vi "state_machine.vi"() -> ()   [LabVIEW 2017, in "DemoSequencer.lvlib"]
uses:
  DemoSequencer.lvlib
  Utilities/WordManipulationLibrary.lvlib
  Utilities/StateMachineStatus.ctl
  Utilities/Bit Manipulation.lvlib
  Utilities/Controlword_Commands.ctl
  Utilities/StateMachine.ctl
panel:
  out "Data Out":u16 format="%08b"
  out "Status":T1
  in  "Device Control Command":T2=enum."Switch On"
  out "Waveform Chart":dbl(graph)
  in  "End Program":bool
  in  "Stop Move":bool
  in  "SLM Velocity":dbl
  in  "SLM Position":dbl
  in  "StraightLineMove":bool
  out "StatusWord":u16
  in  "stop":bool
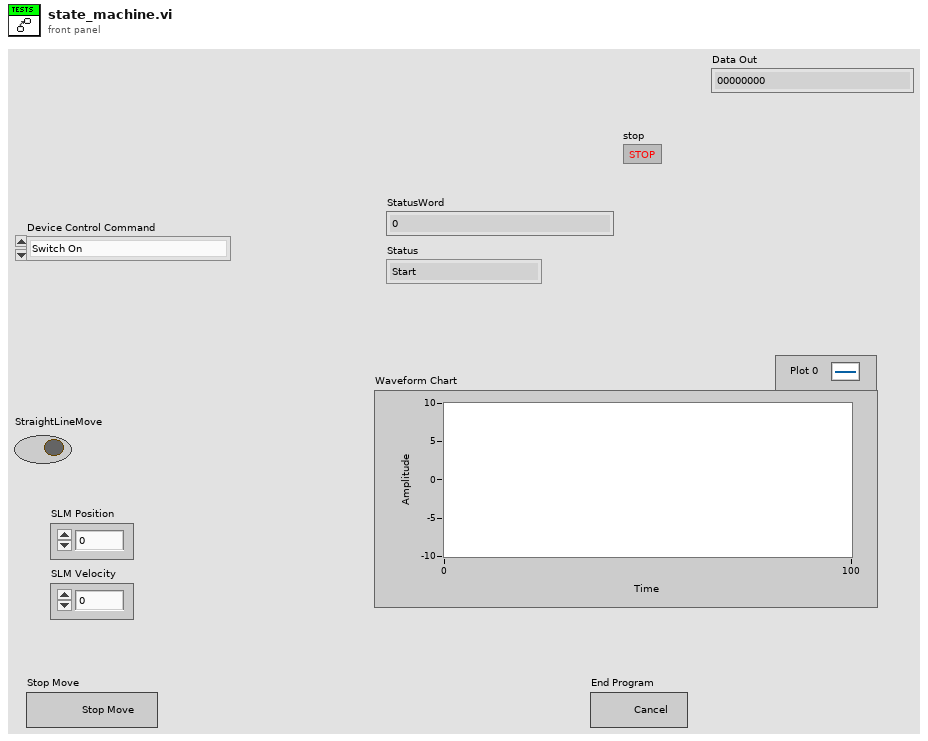
[diagram p1: front panel]
types:
  T1 = typedef "WordManipulationLibrary.lvlib/StateMachine.ctl" = enum16{"Start", "Not Ready to Switch On", "Switch On Disabled", "Ready to Switch On", "Switched On", "Operation enable", "Quick Stop Active", "Fault Reaction Active", "Fault"}
  T2 = typedef "WordManipulationLibrary.lvlib/Controlword_Commands.ctl" = enum16{"Shutdown", "Switch On", "Disable Voltage", "Quick Stop", "Disable Op", "Enable Op", "Fault Reset", "Error"}
  T3 = typedef "StateMachineStatus.ctl" = enum16{"init", "StateMachineManipulation", "waiting", "PreparingMove", "ProcessingMove", "end"}
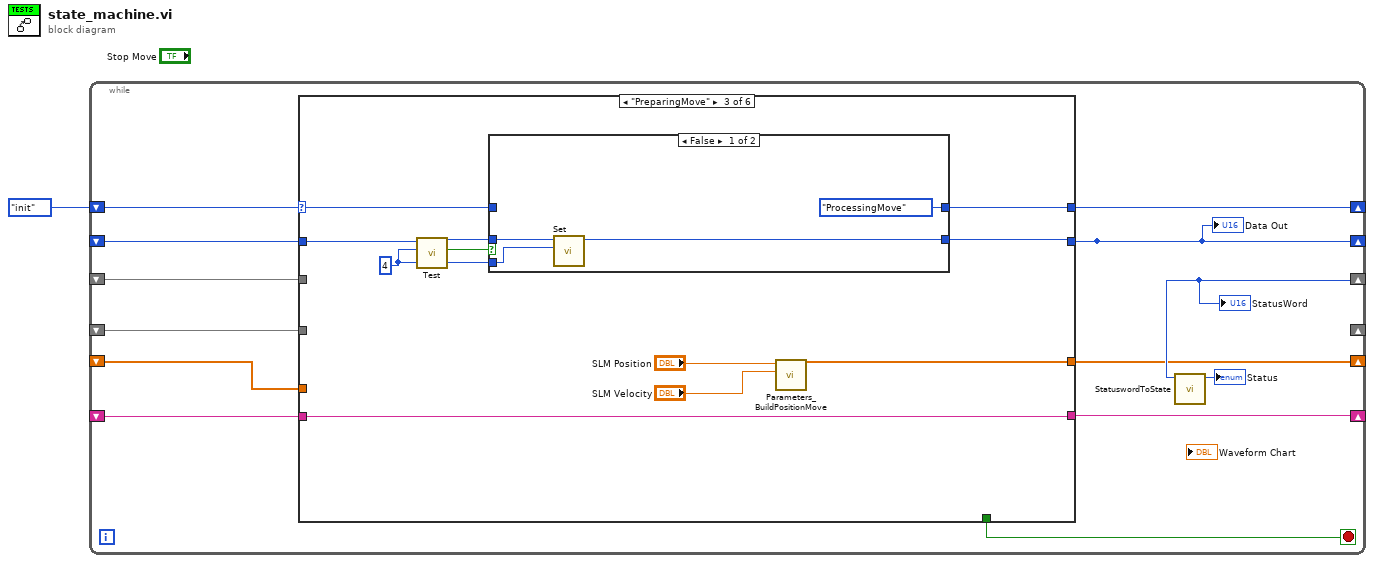
[diagram p0: block diagram]
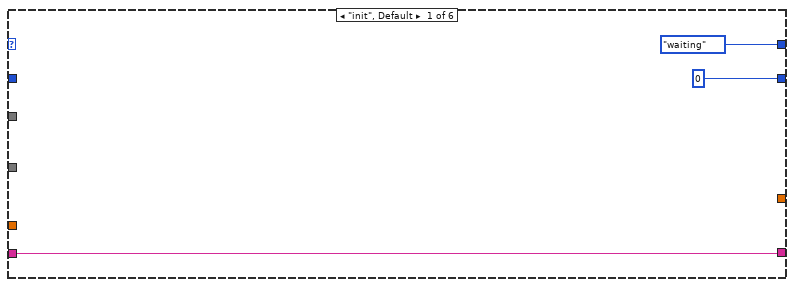
[diagram p2: hidden frame]
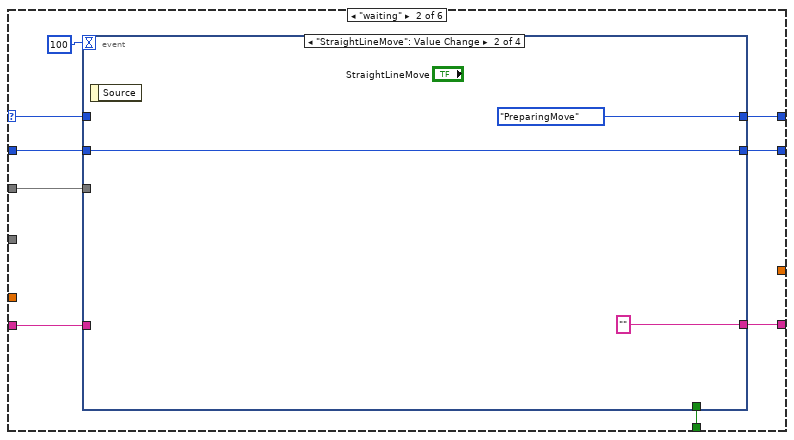
[diagram p3: hidden frame]
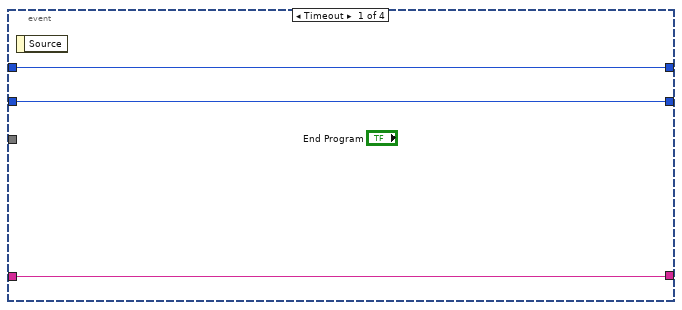
[diagram p4: hidden frame]
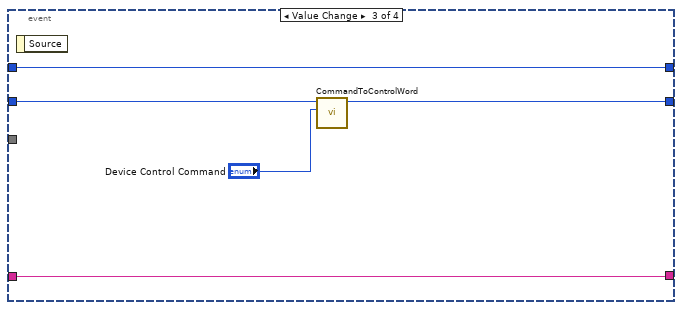
[diagram p5: hidden frame]
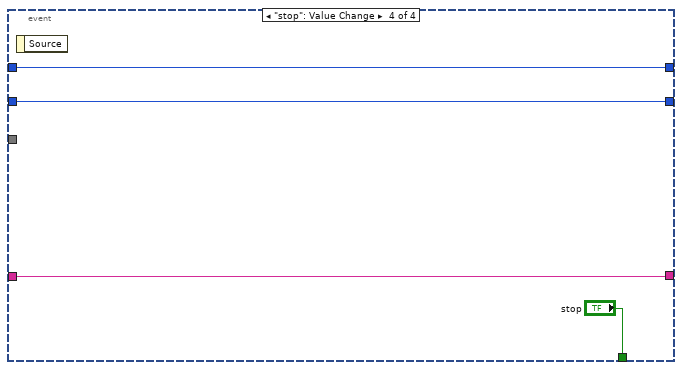
[diagram p6: hidden frame]
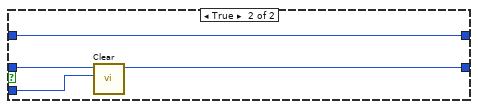
[diagram p7: hidden frame]
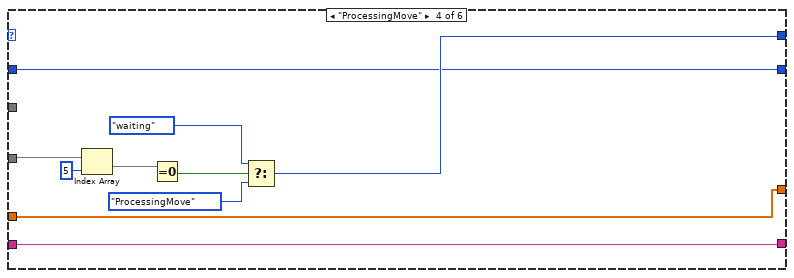
[diagram p8: hidden frame]
diagram:
  n1 = while {
    shift-right: ["StatusWord"] -> _
    shift-left: _ -> [w11]
    shift-right: [w14] -> _
    shift-left: StateMachineStatus."init" -> [w15]
    shift-right: [w13] -> _
    shift-left: _ -> [w12]
    shift-right: [w10] -> _
    shift-left: _ -> [w7]
    shift-right: _ -> [w9]
    shift-left: _ -> [w8]
    shift-right: [w3] -> _
    shift-left: _ -> [w2]
    stop <- w6 stop-if-true
    n2 = case shown="\"PreparingMove\"" w15 {
      selector: w15 -> [_ w23 w47 _ w72 w76]
      tunnel: [u16 0 ("ControlWord") w24 w49 w64 w73 w77] -> w13
      tunnel: [StateMachineStatus."waiting" w22 w48 w65 w72 w76] -> w14
      tunnel: w12 -> [_ w26 w53 w64 w73 w77]
      tunnel: w11 -> [_ w25 _ _ _ _]
      tunnel: [w16 w21 w46 w63 w74 w75] -> w10
      tunnel: [_ _ w43 w62 _ _] -> w3
      tunnel: w8 -> [_ _ _ w71 _ _]
      tunnel: w7 -> [w16 w19 w46 w63 w74 w75]
      tunnel: [_ w20 _ _ _ _] -> w6
      tunnel: w2 -> [_ _ _ w62 _ _]
      frame "init", Default {
      }
      frame "waiting" {
        n3 = event shown="[1] \"StraightLineMove\": Value Change" {
          selector: _ -> [_ _ _ _]
          dyn-events: _ -> [_ _ _ _]
          timeout: 100 -> [_ _ _ _]
          tunnel: w26 -> [w30 w31 w38 w40]
          tunnel: w25 -> [_ _ _ _]
          tunnel: [w30 w31 w36 w40] -> w24
          tunnel: w23 -> [w29 _ w34 w41]
          tunnel: [w29 StateMachineStatus."PreparingMove" w34 w41] -> w22
          tunnel: [w28 "" w35 w39] -> w21
          tunnel: [_ _ _ "stop"] -> w20
          tunnel: w19 -> [w28 _ w35 w39]
          event Timeout {
            n4 = event-data() -> ()  [unwired: 1 in, 1 out]
          }
          event "StraightLineMove": Value Change {
            n5 = event-data() -> ()  [unwired: 1 in, 1 out]
          }
          event Value Change {
            n6 = event-data() -> ()  [unwired: 1 in, 1 out]
            n7 = call "CommandToControlWord.vi"("Device Control Command"="Device Control Command", "ControlWord In"=w38) -> ("ControlWord Out"=w36:u16)  [unwired: 9 in]
          }
          event "stop": Value Change {
            n8 = event-data() -> ()  [unwired: 1 in, 1 out]
          }
        }
      }
      frame "PreparingMove" {
        w50 = u8 4 ("Bit to test")
        n9 = call "Test.vi"("Bit to test"=w50, "Data_In"=w53) -> ("bit value"=w52:bool, "Data_Out"=w51:u16)  [unwired: 8 in]
        n10 = case shown="False" w52 {
          tunnel: w51 -> [w57 w61]
          tunnel: w50 -> [w56 w60]
          tunnel: [w55 w59] -> w49
          tunnel: [StateMachineStatus."ProcessingMove" w58] -> w48
          tunnel: w47 -> [_ w58]
          frame False {
            n11 = call "Set.vi"("Bit to set"=w56, "Data_In"=w57) -> ("Data_Out"=w55:u16)  [unwired: 9 in]
          }
          frame True {
            n12 = call "Clear.vi"("Bit to clear"=w60, "Data_In"=w61) -> ("Data_Out"=w59:u16)  [unwired: 9 in]
          }
        }
        n13 = call "Parameters_BuildPositionMove.vi"("Velocity"="SLM Velocity", "Target Position"="SLM Position") -> ("Parameters"=w43:dbl[])  [unwired: 9 in]
      }
      frame "ProcessingMove" {
        n14 = Index Array(array=w71, index=5) -> (element=w69)
        n15 = Equal To 0?(x=w69) -> (x = 0?=w68:bool)
        n16 = Select(t=StateMachineStatus."waiting", s=w68, f=StateMachineStatus."ProcessingMove") -> (s? t:f=w65:T3)
      }
      frame "end" {
      }
      frame "StateMachineManipulation" {
      }
    }
    "Data Out" <- w13
    n17 = call "StatuswordToState.vi"("Data_In"="StatusWord") -> ("Status"=→"Status":T1)  [unwired: 10 in]
  }
